vi "CRYOpen Step.vi"(11 "Step No.":u16) -> ()   [LabVIEW 2013]
uses:
  CRYProject Editor Global.vi
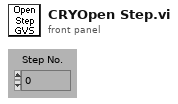
[diagram p1: front panel]
types:
  T1 = typedef "CRYTS.ctl" = cluster{"No.TS":u16, "TS File Path":path, "TS Name":string, "EditStepName":string, "Steps":T2[], "New State":bool, "Change State":bool, "Flattened CurveLib Data":string, "Document Data":string, "EditStepNo":u16, "Operator Start File":string, "Sequence Type":string, "Sequence Language":string}
  T2 = typedef "CRYStep.ctl" = cluster{"No.VI":i32, "Category":string, "StepName":string, "Seq setup flattened":string, "Comment":string, "Steps config.":bool[], "Jump config":i32[], "Start":dbl, "Increment":dbl, "Name":string, "Unit":string, "Y data":u16, "Y prefix":string, "Y dB ref":dbl, "Y unit":string, "Repeat State Array":cluster{"Start":dbl, "Increment":dbl, "Count":i32, "Num":i32}[]}
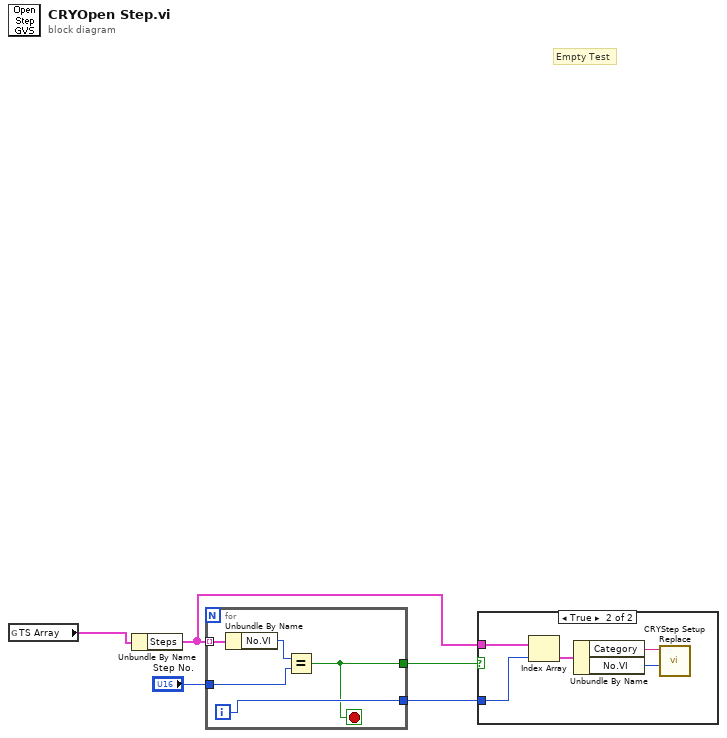
[diagram p0: block diagram]
diagram:
  # "Empty Test"
  n1 = global read "CRYProject Editor Global.vi" "TS Array"() -> (w1:T1)
  n2 = Unbundle By Name(w1) -> ("Steps"=w4:T2[])
  n3 = for {
    tunnel: w4 -> [w10] mode=indexing
    tunnel: "Step No." -> [w8]
    tunnel: [w7] -> w3
    tunnel: [w6] -> w2
    i -> [w7]
    stop <- w6 stop-if-true
    n4 = Unbundle By Name(w10) -> ("No.VI"=w9:i32)
    n5 = Equal?(x=w9, y=w8) -> (x = y?=w6:bool)
  }
  n6 = case shown="True" w2 {
    tunnel: w4 -> [_ w12]
    tunnel: w3 -> [_ w11]
    frame False {
    }
    frame True {
      n7 = Index Array(array=w12, index=w11) -> (element=w14:T2)
      n8 = Unbundle By Name(w14) -> ("Category"=w15:string, "No.VI"=w13:i32)
      n9 = call "CRYStep Setup Replace.vi"("Current Step Setup VI No"=w13, "Category"=w15) -> ()  [unwired: 2 in, 8 out]
    }
  }
